vi "GetGObjects_BD.vi"(8 "error in":errorcluster, 11 "VI Interpreter in":refnum<class "VI Interpreter.lvclass">) -> (0 "error out":errorcluster, 3 "VI Interpreter out":refnum<class "VI Interpreter.lvclass">)   [LabVIEW 2014, in "VI Interpreter.lvclass"]
uses:
  VI Interpreter.lvclass
  VI Interpreter.lvclass/VI Interpreter.ctl
  <vilib>/Utility/traverseref.llb/TRef TravTarget.ctl
  GObject/GObject.lvclass
  <vilib>/Utility/traverseref.llb/VI Scripting - Traverse.lvlib
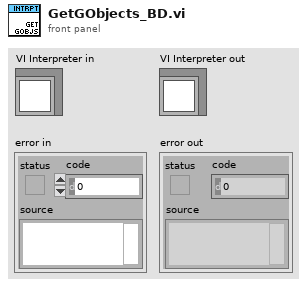
[diagram p1: front panel]
types:
  T1 = typedef "TRef TravTarget.ctl" = enum16{"FP", "BD", "Other"}
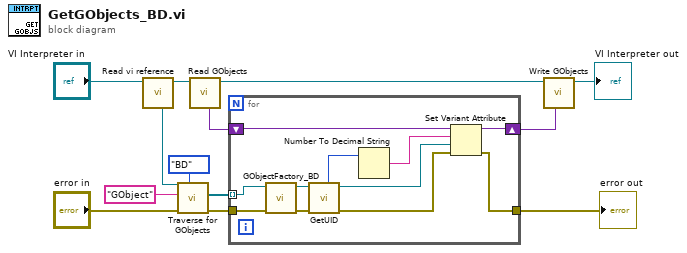
[diagram p0: block diagram]
diagram:
  n1 = call "Read vi reference.vi"("VI Interpreter in"="VI Interpreter in") -> ("VI Interpreter out"=w3:refnum<class "VI Interpreter.lvclass">, "vi reference"=w8:refnum<vi>)  [unwired: 7 in]
  n2 = call <vilib>:"Traverse for GObjects.vi"("Traverse Target"=TRef_TravTarget."BD", "error in (no error)"="error in", "Class Name"="GObject", "VI Refnum"=w8) -> ("error out"=w12:errorcluster, "References"=w11:refnum<vi>[])  [unwired: 4 in, 2 out]
  n3 = call "Read GObjects.vi"("VI Interpreter in"=w3) -> ("VI Interpreter out"=w2:refnum<class "VI Interpreter.lvclass">, "GObjects"=w1:variant)  [unwired: 7 in]
  n4 = for {
    tunnel: w11 -> [w14] mode=indexing
    shift-right: [w24] -> w5
    shift-left: w1 -> [w23]
    tunnel: w12 -> [w15]
    tunnel: [w21] -> w6
    n5 = call "GObjectFactory_BD.vi"("error in"=w15, "reference"=w14) -> ("error out"=w16:errorcluster, "GObject out"=w17:refnum<class "GObject.lvclass">)  [unwired: 8 in]
    n6 = call-dynamic "GetUID.vi"("error in"=w16, "GObject in"=w17) -> ("error out"=w18:errorcluster, "GObject out"=w19:refnum<class "GObject.lvclass">, "UID"=w20:i32)  [unwired: 5 in]
    n7 = Number To Decimal String(number=w20) -> (decimal integer string=w22:string)  [unwired: 1 in]
    n8 = Set Variant Attribute(Variant=w23, name=w22, value=w19, error in=w18) -> (Variant out=w24:variant, error out=w21:errorcluster)  [unwired: 1 out]
  }
  "error out" <- w6
  n9 = call "Write GObjects.vi"("GObjects"=w5, "VI Interpreter in"=w2) -> ("VI Interpreter out"=→"VI Interpreter out":refnum<class "VI Interpreter.lvclass">)  [unwired: 7 in]
